vi "Board Display.vi"(8 "error in (no error)":errorcluster, 11 "Board in":refnum<class "Board.lvclass">) -> (0 "error out":errorcluster, 2 "2D Picture Out":picture, 3 "Board out":refnum<class "Board.lvclass">)   [LabVIEW 2019, in "Board.lvclass"]
uses:
  Board.lvclass
  Food/Food.lvclass
  Player/Player.lvclass
  Snake/Snake.lvclass
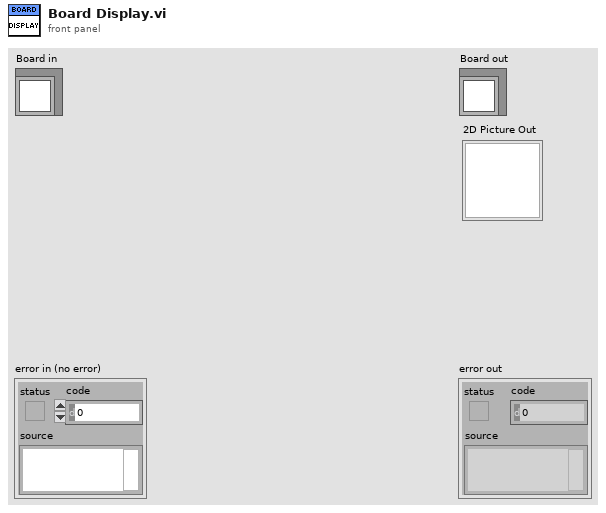
[diagram p1: front panel]
types:
  T1 = typedef "Coordinate STYP.ctl" = cluster{"X":i32, "Y":i32}
  T2 = cluster{"left":i16, "top":i16, "right":i16, "bottom":i16}
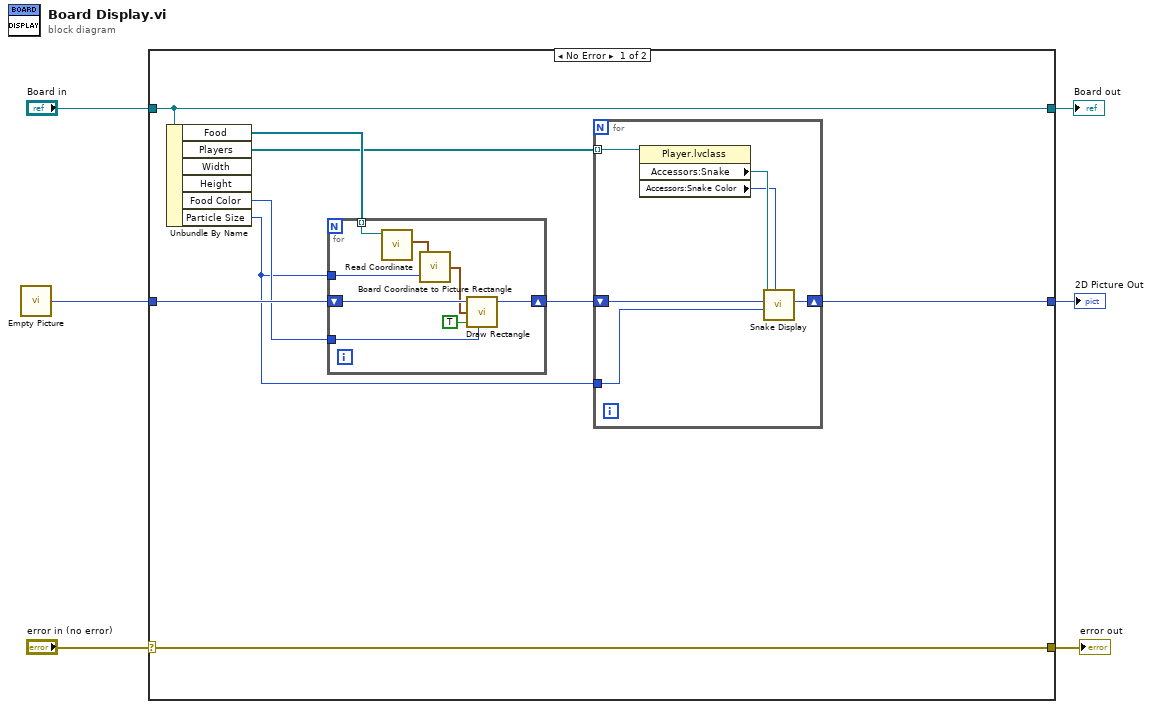
[diagram p0: block diagram]
diagram:
  n1 = call "Empty Picture"() -> ("empty picture"=w2:picture)
  n2 = case shown="No Error" "error in (no error)" {
    selector: "error in (no error)" -> [w15 w31]
    tunnel: [w15 w31] -> w5
    tunnel: [w14 w30] -> w3
    tunnel: "Board in" -> [w14 w30]
    tunnel: w2 -> [w12 _]
    tunnel: [w8 _] -> w1
    frame No Error {
      n3 = Unbundle By Name(w14) -> ("Food"=w13:refnum<class "Food.lvclass">[], "Players"=w10:refnum<class "Player.lvclass">[], "Food Color"=w11:u32, "Particle Size"=w7:u32)  [unwired: 2 out]
      n4 = for {
        tunnel: w13 -> [w29] mode=indexing
        tunnel: w7 -> [w27]
        shift-right: [w22] -> w9
        shift-left: w12 -> [w26]
        tunnel: w11 -> [w23]
        n5 = call-dynamic "Read Coordinate.vi"("Food in"=w29) -> ("Coordinate"=w28:T1)  [unwired: 8 in, 2 out]
        n6 = call "Board Coordinate to Picture Rectangle.vi"("Particle Size"=w27, "Coordinate"=w28) -> ("rect"=w25:T2)
        n7 = call <vilib>:"Draw Rectangle.vi"("picture"=w26, "rect"=w25, "fill?(F)"=TRUE, "color(black)"=w23) -> ("new picture"=w22:picture)  [unwired: 5 in]
      }
      n8 = for {
        tunnel: w10 -> [w21] mode=indexing
        shift-right: [w17] -> w8
        shift-left: w9 -> [w18]
        tunnel: w7 -> [w16]
        n9 = property class="Player.lvclass"(reference=w21) -> ("Accessors:Snake"=w20:refnum<class "Snake.lvclass">, "Accessors:Snake Color"=w19:u32)  [unwired: 1 in, 2 out]
        n10 = call-dynamic "Snake Display.vi"("Color"=w19, "Particle Size"=w16, "2D Picture"=w18, "Snake in"=w20) -> ("2D Picture Out"=w17:picture)  [unwired: 5 in, 2 out]
      }
    }
    frame Error {
    }
  }
  "error out" <- w5
  "Board out" <- w3
  "2D Picture Out" <- w1
